vi "ReadWriteInputOutput.vi"(8 "Input Index":i32[](array[numeric]), 9 "Output Index":i32[](array[numeric]), 10 "Inputs":bool[](array[boolean]), 11 "data table in":T1) -> (2 "Outputs":bool[](array[boolean]), 3 "data table out":T1)   [LabVIEW 2013]
uses:
  <vilib>/NI/Tag Bus/table/data table.ctl
  <vilib>/NI/Tag Bus/table/data polymorphs/write one/write Boolean.vi
  <vilib>/NI/Tag Bus/table/data polymorphs/read one/read Boolean.vi
  <vilib>/NI/Tag Bus/table/data table.lvlib
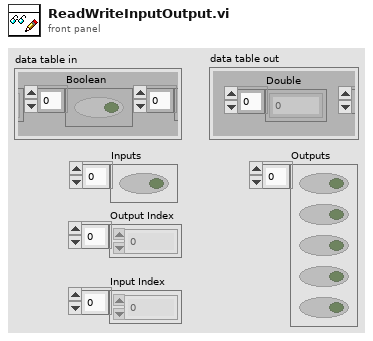
[diagram p1: front panel]
types:
  T1 = typedef "tag bus.lvlib/data table.lvlib/data table.ctl" = cluster{"Double":dbl[], "Single":sgl[], "I64":i64[], "I32":i32[], "I16":i16[], "I8":i8[], "U64":u64[], "U32":u32[], "U16":u16[], "U8":u8[], "Boolean":bool[], "String":string[], "Array of Double":cluster{"DBL Array":dbl[]}[], "Array of Single":cluster{"SGL Array":sgl[]}[], "Array of I64":cluster{"I64 Array":i64[]}[], "Array of I32":cluster{"I32 Array":i32[]}[], "Array of I16":cluster{"I16 Array":i16[]}[], "Array of I8":cluster{"I8 Array":i8[]}[], "Array of U64":cluster{"U64 Array":u64[]}[], "Array of U32":cluster{"U32 Array":u32[]}[], "Array of U16":cluster{"U16 Array":u16[]}[], "Array of U8":cluster{"U8 Array":u8[]}[], "Array of Boolean":cluster{"Boolean Array":bool[]}[], "Array of String":cluster{"String Array":string[]}[]}
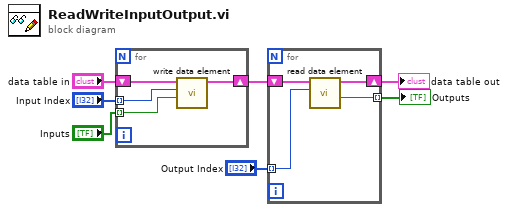
[diagram p0: block diagram]
diagram:
  n1 = for {
    shift-right: [w11] -> w2
    shift-left: "data table in" -> [w10]
    tunnel: "Input Index" -> [w9] mode=indexing
    tunnel: "Inputs" -> [w8] mode=indexing
    n2 = call-poly <vilib>:"write data element.vi"("value"=w8, "index"=w9, "data table in"=w10) -> ("data table out"=w11:T1)  [unwired: 8 in]
  }
  n3 = for {
    shift-right: [w13] -> w1
    shift-left: w2 -> [w15]
    tunnel: "Output Index" -> [w14] mode=indexing
    tunnel: [w12] -> w5 mode=indexing
    n4 = call-poly <vilib>:"read data element.vi"("index"=w14, "data table in"=w15) -> ("value"=w12:bool, "data table out"=w13:T1)  [unwired: 8 in]
  }
  "data table out" <- w1
  "Outputs" <- w5
